vi "TEDS Binary to Table.vi"(3 "error in":errorcluster, 4 "v0.9 TEDS (F)":bool, 5 "template file directory":path, 6 "TEDS Binary":bool[](array[boolean])) -> (0 "error out":errorcluster, 1 "TEDS":T1={"TEDS Error?"=FALSE, "TEDS Error"=" INSTRUCTIONS:\r\rNormal Use:  When using subVIs that incorporate the error in/error out (or error I/O) structure, place this handler where you want to inform the user of an error, typically at the end of the I/O data path, as the last action of the program.  If the error in error? is ERROR, the handler creates a message describing the error and its source.  If the type of dialog = 1 (default), the message is displayed to the user, who can only acknowedge it.  If the type = 2, the user can acknowledge the message or abort execution; aborting a program with active I/O is not recommended.  If the type = 0, no message is displayed; this is used to process the error programmatically, and the error out cluster elements are wired to individual terminals for that reason.  \r\rOther Use:\n\r\nlocal testing.  To test the error code of a subVI or function that does not have the error I/O structure, you can wire its error code and a source string to the local error code and error source inputs.  If error in error? indicates no error and error code is not equal to 0, the local code and source are substituted for the error in values, and error? is set TRUE (ERROR).", "TEDS Data"=[]})   [LabVIEW 2021]
uses:
  <vilib>/Utility/error.llb/DialogType.ctl
  Program Files/National Instruments/LabVIEW 2021/vi.lib/teds/TEDS_api.llb/TEDS_Parse Binary TEDS.vi
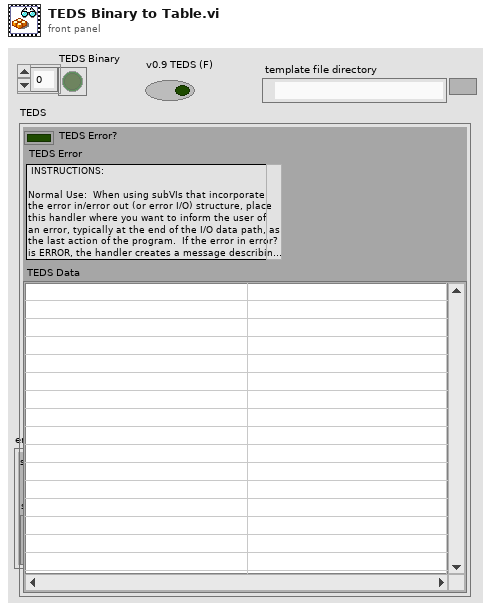
[diagram p1: front panel]
types:
  T1 = cluster{"TEDS Error?":bool, "TEDS Error":string, "TEDS Data":string[][]}
  T2 = typedef "teds_Line and Bits.ctl" = cluster{"Line":string[], "Bits":bool[]}
  T3 = typedef "DialogType.ctl" = u16
  T4 = cluster{bool, "message":string, "table":string[][]}
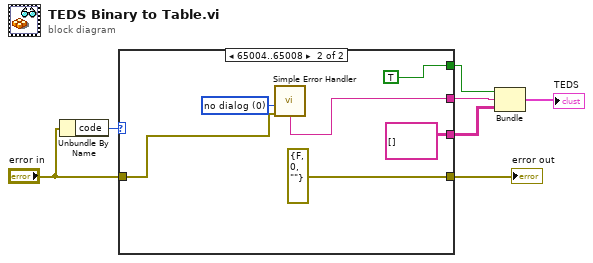
[diagram p0: block diagram]
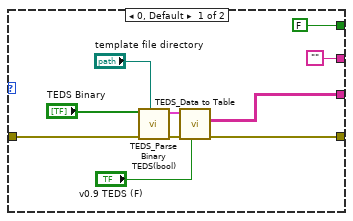
[diagram p2: hidden frame]
diagram:
  n1 = Unbundle By Name("error in") -> ("code"=w6:i32)
  n2 = case shown="65004..65008" w6 {
    tunnel: "error in" -> [w10 w20]
    tunnel: [FALSE TRUE] -> w4
    tunnel: ["" w19] -> w3
    tunnel: [w9 errorcluster {"status"=FALSE, "code"=0, "source"=""} ("error in")] -> w5
    tunnel: [w8 string[][] [] ("table")] -> w2
    frame 0, Default {
      n3 = call-poly "TEDS_Parse Binary TEDS(bool).vi"("template file directory"="template file directory", "error in (no error)"=w10, "binary TEDS array"="TEDS Binary") -> ("error out"=w13:errorcluster, "TEDS data out"=w12:T2[])  [unwired: 7 out]
      n4 = call "TEDS_Data to Table.vi"("v0.9 TEDS (F)"="v0.9 TEDS (F)", "error in (no error)"=w13, "TEDS data in"=w12) -> ("error out"=w9:errorcluster, "table"=w8:string[][])  [unwired: 7 out]
    }
    frame 65004..65008 {
      w18 = T3 0 items=["no dialog", "OK message", "continue or stop message", "OK message + warnings", "continue/stop + warnings"] ("type of dialog (OK msg:1)")
      n5 = call <vilib>:"Simple Error Handler.vi"("type of dialog (OK msg:1)"=w18, "error in (no error)"=w20) -> ("message"=w19:string)  [unwired: 7 out]
    }
  }
  "error out" <- w5
  n6 = Bundle(w4, "message"=w3, "table"=w2) -> (→"TEDS":T4)  [unwired: 1 out]
